vi "Reserve Callback.vi"(8 "error in":errorcluster, 10 "session infos":T1[](array[typedef]), 11 "measurement context in":refnum<class "Measure Call Context.lvclass">) -> (0 "error out":errorcluster, 3 "measurement context out":refnum<class "Measure Call Context.lvclass">)   [LabVIEW 2020, in "Plug-In SDK Measurement.lvlib" / "Measure Call Context.lvclass"]
uses:
  Measure Call Context.lvclass
  gRPC/Generated APIs/ni/measurementlink/sessionmanagement/v1/RPC Messages/ni_measurementlink_sessionmanagement_v1_SessionInformation.ctl
  gRPC/Generated APIs/ni/measurementlink/sessionmanagement/v1/RPC Messages/nidevice_grpc_Session.ctl
  gRPC/Generated APIs/ni/measurementlink/sessionmanagement/v1/RPC Messages/ni_measurementlink_sessionmanagement_v1_ChannelMapping.ctl
  Measure Call Context.lvclass/Measure Call Context.ctl
  gRPC/Generated APIs/ni/measurementlink/sessionmanagement/v1/ni.measurementlink.sessionmanagement.v1.lvlib
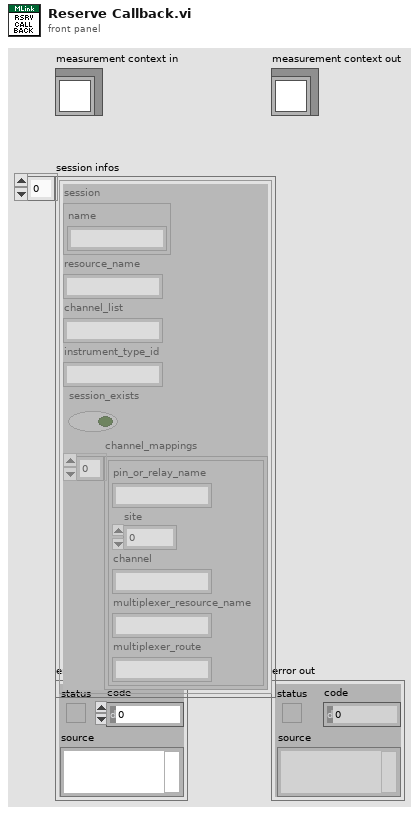
[diagram p1: front panel]
types:
  T1 = typedef "ni.measurementlink.sessionmanagement.v1.lvlib/ni_measurementlink_sessionmanagement_v1_SessionInformation.ctl" = cluster{"session":T2, "resource_name":string, "channel_list":string, "instrument_type_id":string, "session_exists":bool, "channel_mappings":T3[]}
  T2 = typedef "ni.measurementlink.sessionmanagement.v1.lvlib/nidevice_grpc_Session.ctl" = cluster{"name":string}
  T3 = typedef "ni.measurementlink.sessionmanagement.v1.lvlib/ni_measurementlink_sessionmanagement_v1_ChannelMapping.ctl" = cluster{"pin_or_relay_name":string, "site":i32, "channel":string, "multiplexer_resource_name":string, "multiplexer_route":string}
  T4 = typedef "Plug-In SDK Measurement.lvlib/Measure Call Context.lvclass/Data.ctl" = cluster{"pin map context":T5, "gRPC ID":T6, "measurement service":refnum<class "IMeasurement Service.lvclass">, "measurement plugin service":refnum<class "Measurement Plugin Service.lvclass">, "reserved session infos":set{T1}}
  T5 = typedef "Plug-In SDK Measurement.lvlib/Pin Map Context.ctl" = cluster{"pin map id":string, "sites":i32[]}
  T6 = typedef "grpc-lvsupport-release.lvlib/grpcId.ctl" = u64
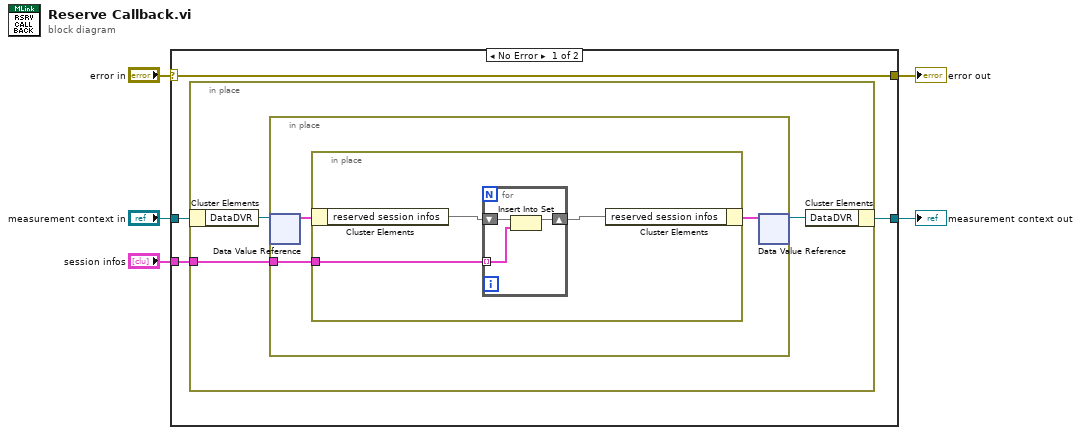
[diagram p0: block diagram]
diagram:
  n1 = case shown="No Error" "error in" {
    selector: "error in" -> [w6 w23]
    tunnel: "measurement context in" -> [w9 w22]
    tunnel: [w8 w22] -> w4
    tunnel: "session infos" -> [w7 _]
    tunnel: [w6 w23] -> w1
    frame No Error {
      n2 = in-place {
        in-place-border: w7 -> [w10]
        n3 = in-place-cluster #1(w9) -> ("DataDVR"=w12:refnum<data-value>)
        n4 = in-place {
          in-place-border: w10 -> [w13]
          n5 = in-place-dvr #2(w12) -> (w15:T4)  [unwired: 1 out]
          n6 = in-place {
            in-place-border: w13 -> [w16]
            n7 = in-place-cluster #3(w15) -> ("reserved session infos"=w18:set{T1})
            n8 = for {
              tunnel: w16 -> [w19] mode=indexing
              shift-right: [w20] -> w17
              shift-left: w18 -> [w21]
              n9 = Insert Into Set(10:w19, 11:w21) -> (3:w20:set{T1})  [unwired: 1 out]
            }
            n10 = in-place-cluster #3("reserved session infos"=w17) -> (w14:T4)
          }
          n11 = in-place-dvr #2(w14) -> (w11:refnum<data-value>)  [unwired: 1 out]
        }
        n12 = in-place-cluster #1("DataDVR"=w11) -> (w8:refnum<class "Measure Call Context.lvclass">)
      }
    }
    frame Error {
    }
  }
  "error out" <- w1
  "measurement context out" <- w4
